vi "HOG Main.vi"() -> ()   [LabVIEW 2018]
doc: "This template is for the Queued Message Handler design pattern.\n\nThe Event Handling Loop generates messages based on user interface actions.\n\nThe Message Handling Loop processes messages generated by the Event Handling Loop, or by other messages. The messages are string values, so new messages can be added easily to the Message Cases case structure in the Message Handling Loop. Each message cluster can also provide an optional value for Message Data, which is a variant that can be converted to whatever message-specific data is required."
uses:
  controls/HOG UI Data.ctl
  <vilib>/GPower/Logger - Text/Library/Text Logger Class/Text Logger.lvclass
  C:/Program Files (x86)/National Instruments/LabVIEW 2018/vi.lib/GPower/Logger/Library/Logger Class/Logger.lvclass
  <vilib>/GPower/Dictionary/Library/Dictionary Class/Dictionary.lvclass
  support/Diploma Info.ctl
  <vilib>/Utility/sysdir.llb/System Directory Type.ctl
  <vilib>/GPower/Logger/Library/Logger Class/Logger.lvclass/Logger.ctl
  <vilib>/GPower/Array/Library/SearchMult/SearchMult1.vi
  8841ee87-444d-4723-9e2d-6f9928da492d.vi
  <vilib>/GPower/Logger/Library/Logger Class/Accessors/Get Enabled State.vi
  <vilib>/GPower/Logger/Library/Logger Class/Accessors/Get Severity Level Threshold.vi
  <vilib>/GPower/Logger/Library/Logger Class/Logger/Promote.vi
  <vilib>/GPower/Logger/Library/Logger Class/Accessors/Get Error And Warning Promotion.vi
  support/Message Queue/Enqueue Message (Single).vi
  <vilib>/GPower/Dictionary/Library/Dictionary Class/Get/Get Path.vi
  <vilib>/Utility/error.llb/Error Cluster From Error Code.vi
  <vilib>/GPower/UI/Library/Controls/Clear Control/Clear Listbox.vi
  <vilib>/GPower/UI/Library/Redraw/Defer Panel Updates (VI).vi
  <vilib>/GPower/UI/Library/Redraw/Undefer Panel Updates (VI).vi
  <vilib>/ErrorRing/Error Ring.xnode
  <vilib>/GPower/Logger/Library/Logger Class/Logger.lvclass
  support/Message Queue/HOG Message Queue.lvlib
  support/User Event - Stop/HOG User Event - Stop.lvlib
  <vilib>/GPower/UI/Library/GP UI.lvlib
  <vilib>/GPower/Array/GPArray.lvlib
  <vilib>/GPower/String/Library/GPString.lvlib
  <vilib>/Utility/NIReport.llb/NI_ReportGenerationCore.lvlib
  <vilib>/GPower/Files & Folders/Library/GPFilesFolders.lvlib
panel:
  in  "Tab Control":enum32{"Page 1", "Page 2", "Page 3"}(tab)
  in  "Load Event":bool
  in  "Event Folder Path":path
  in  "Manual":bool
  in  "MemberList":i32[](listbox)
  in  "Search":string
  out "Status":string
  in  "Cancel Print":bool
  in  "Print Button":bool
  in  "Help Radio Buttons":enum32{"Help", "No Help"}(radio) caption="Hjælpemiddel?"
  out "Diplom Navn":string
  out "Længde":string
  out "Diplom Pitcture":u16(ring)
  in  "Length Radio Buttons":enum32{"Baner", "Længde"}(radio)
  in  "Baner":u16
  in  "Navn":string
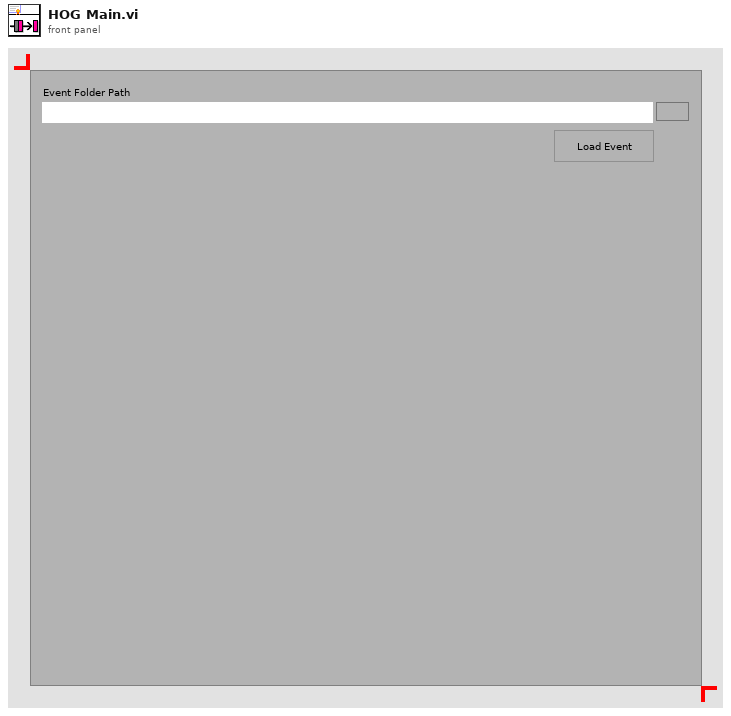
[diagram p1: front panel]
types:
  T1 = typedef "HOG UI Data.ctl" = cluster{"Status Ref":refnum<vi>, "Exit Button Ref":refnum<vi>, "Search Ref":refnum<vi>, "MemberList Ref":refnum<vi>, "This VI Ref":refnum<vi>, "Event Folder Path":path, "Load Event Ref":refnum<vi>, "Tab Control Ref":refnum<vi>, "Baner Ref":refnum<vi>, "Printer Name":string, "Diploma Template Path":path, "Text Logger":refnum<class "Text Logger.lvclass">}
  T2 = typedef "HOG Message Queue.lvlib/All Message Queues.ctl" = cluster{"UI":refnum<queue>, "Member":refnum<queue>}
  T3 = typedef "Diploma Info.ctl" = cluster{"Name":string, "Length Diploma":string, "Length":u16, "Help?":bool}
  T4 = typedef "System Directory Type.ctl" = i32
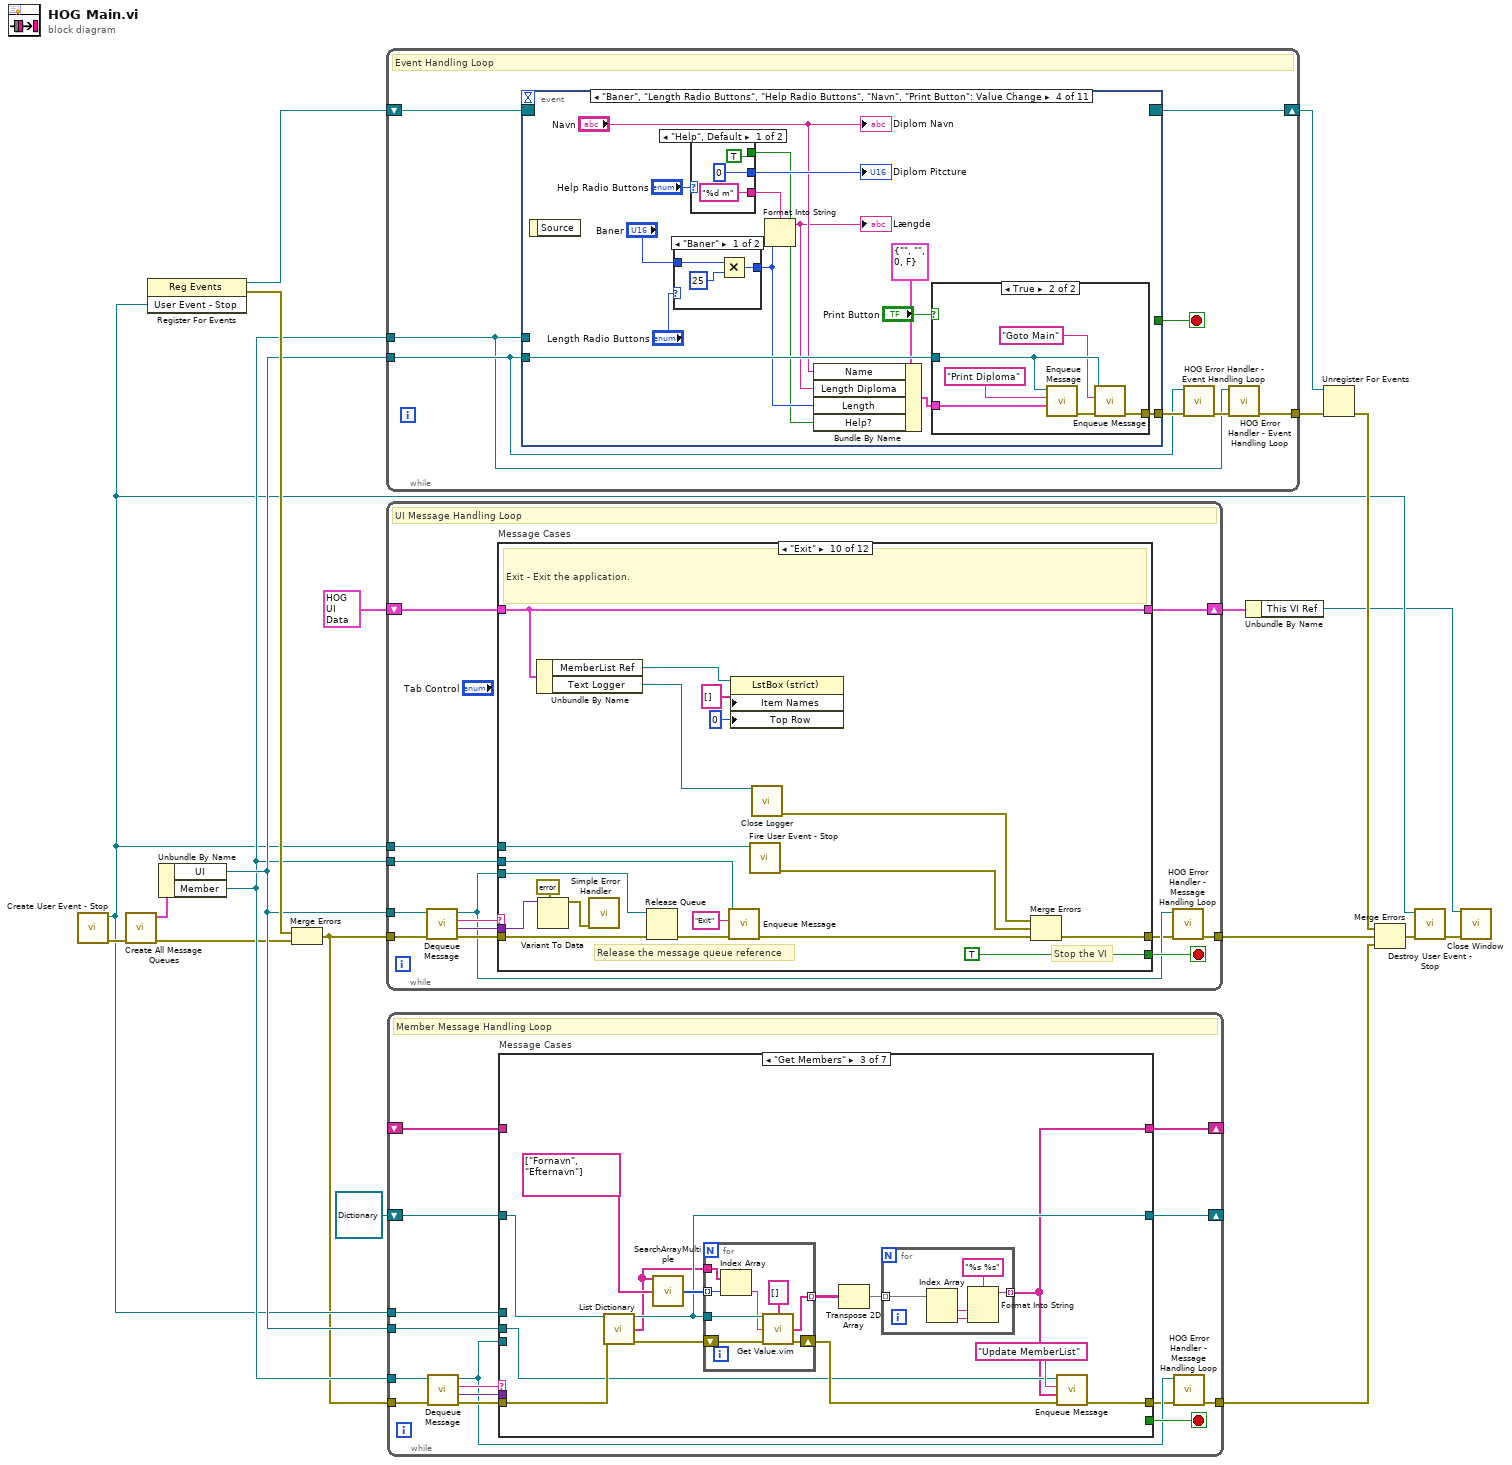
[diagram p0: block diagram]
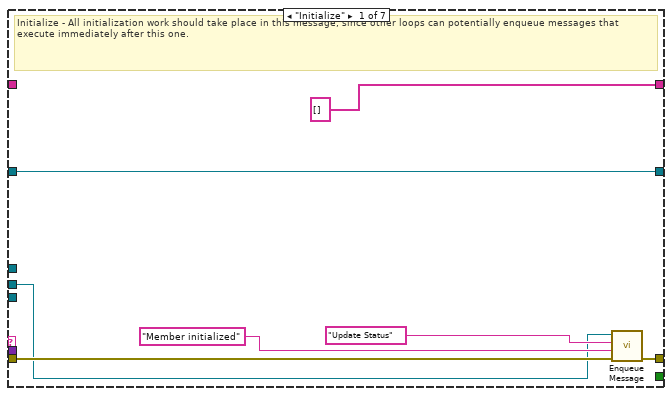
[diagram p2: hidden frame]
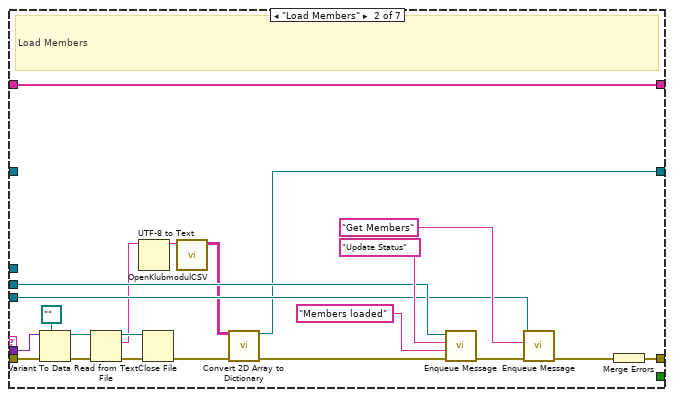
[diagram p3: hidden frame]
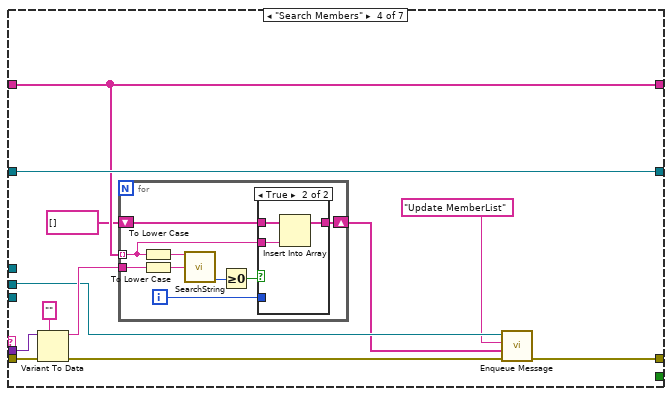
[diagram p4: hidden frame]
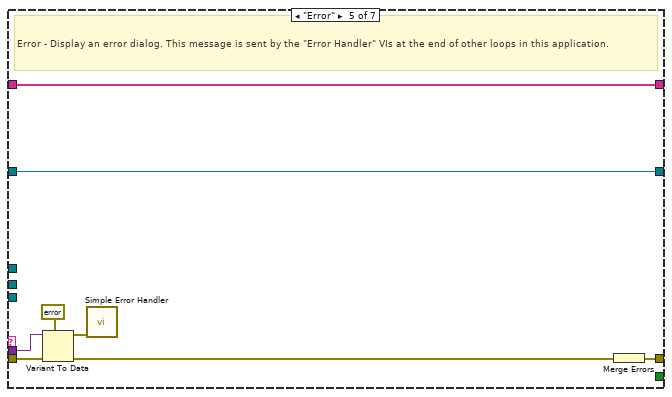
[diagram p6: hidden frame]
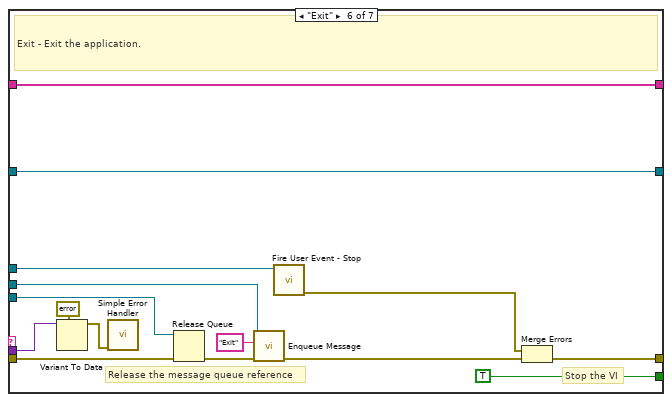
[diagram p7: hidden frame]
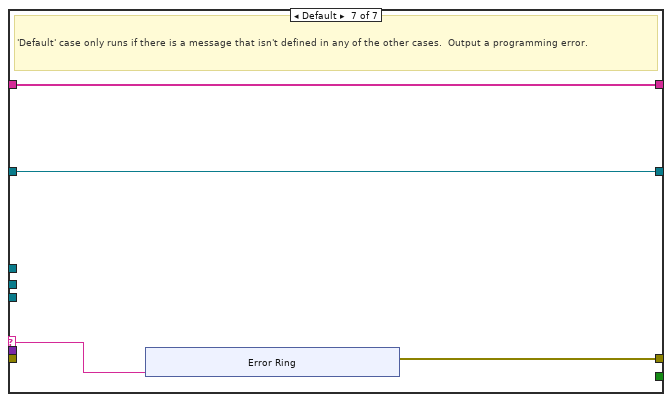
[diagram p8: hidden frame]
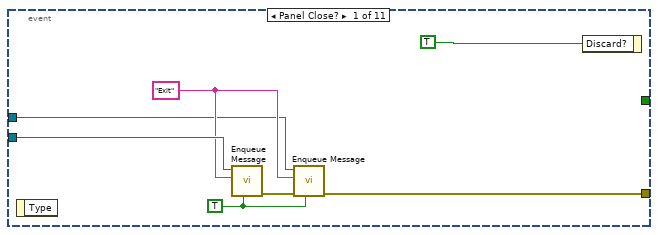
[diagram p9: hidden frame]
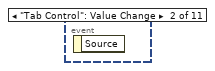
[diagram p10: hidden frame]
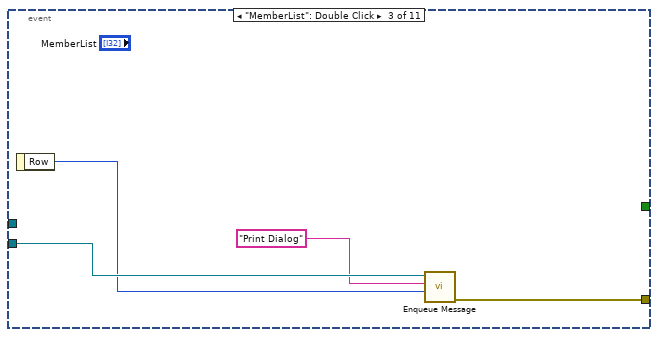
[diagram p11: hidden frame]
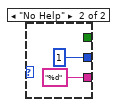
[diagram p14: hidden frame]
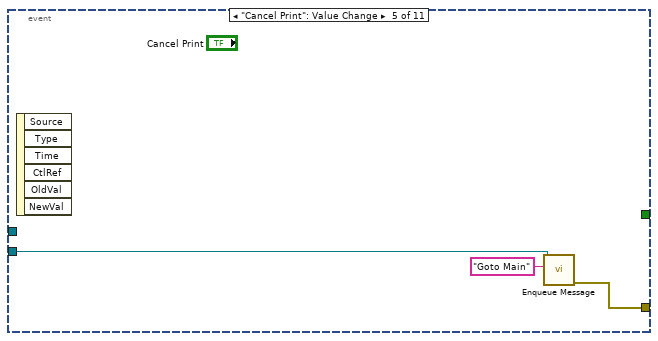
[diagram p15: hidden frame]
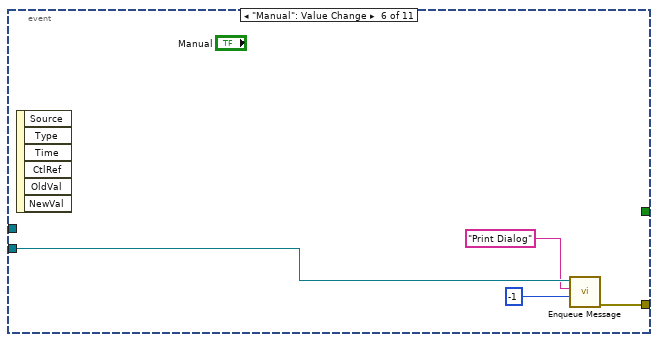
[diagram p16: hidden frame]
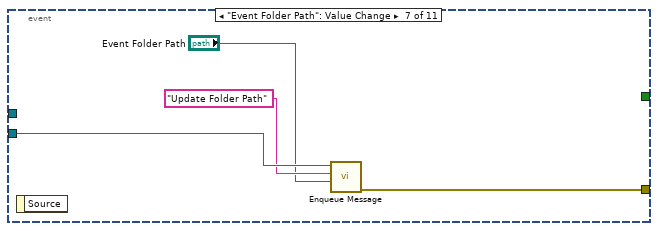
[diagram p17: hidden frame]
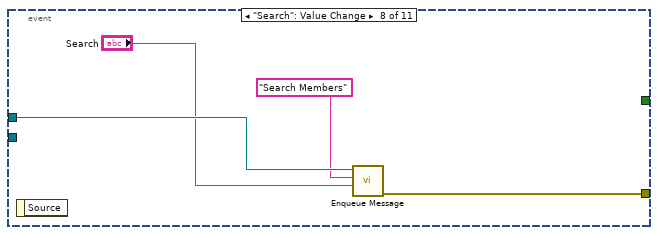
[diagram p18: hidden frame]
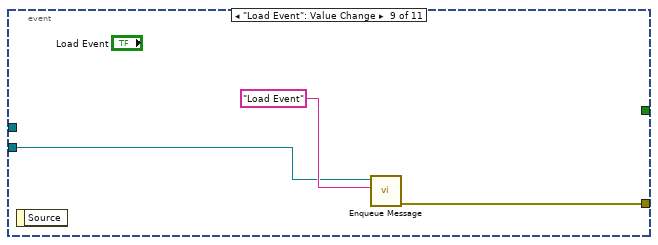
[diagram p19: hidden frame]
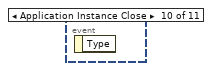
[diagram p20: hidden frame]
diagram:
  n1 = call "Create User Event - Stop.vi"() -> ("error out"=w18:errorcluster, "User Event - Stop"=w6:refnum<user-event>)  [unwired: 10 in]
  n2 = call "Create All Message Queues.vi"("error in (no error)"=w18) -> ("error out"=w5:errorcluster, "Message Queues out"=w20:T2)  [unwired: 9 in]
  n3 = register-events(w6) -> (reference out=w12:refnum<event-registration>, error out=w11:errorcluster)  [unwired: 2 in]
  n4 = Unbundle By Name(w20) -> ("UI"=w9:refnum<queue>, "Member"=w7:refnum<queue>)
  n5 = Merge Errors(w11, w5) -> (w4:errorcluster)
  n6 = while {
    tunnel: w9 -> [w22]
    shift-right: [w27] -> w15
    shift-left: w12 -> [w28]
    tunnel: [w23] -> w13
    tunnel: w7 -> [w21]
    stop <- w25 stop-if-true
    # "Event Handling Loop"
    n7 = event shown="[3] \"Baner\", \"Length Radio Buttons\", \"Help Radio Buttons\", \"Navn\", \"Print Button\": Value Change" {
      selector: w28 -> [_ _ _ _ _ _ _ _ _ _ _]
      dyn-events: [_ _ _ _ _ _ _ _ _ _ _] -> w27
      timeout: _ -> [_ _ _ _ _ _ _ _ _ _ _]
      tunnel: [_ _ _ _ _ _ _ _ _ _ TRUE ("Discard?")] -> w25
      tunnel: w22 -> [w34 _ w38 w50 w70 w74 w78 _ w84 _ _]
      tunnel: [w32 _ w39 w49 w71 w75 w79 w83 w86 _ _] -> w26
      tunnel: w21 -> [w30 _ _ _ _ _ _ w82 _ _ _]
      event Panel Close? {
        w29 = TRUE ("Priority Message? (F)")
        w31 = "Exit" ("Message")
        n8 = event-data() -> ()  [unwired: 1 in, 1 out]
        n9 = call-poly "Enqueue Message.vi"("Priority Message? (F)"=w29, "Message"=w31, "Message Queue"=w34) -> ("error out"=w33:errorcluster)  [unwired: 7 in, 1 out]
        n10 = call-poly "Enqueue Message.vi"("Priority Message? (F)"=w29, "error in (no error)"=w33, "Message"=w31, "Message Queue"=w30) -> ("error out"=w32:errorcluster)  [unwired: 6 in, 1 out]
        n11 = event-data("Discard?"=TRUE) -> ()  [unwired: 1 in, 1 out]
      }
      event "Tab Control": Value Change {
        n12 = event-data() -> ()  [unwired: 1 in, 1 out]
      }
      event "MemberList": Double Click {
        n13 = event-data() -> ("Row"=w36:i32)  [unwired: 1 in]
        n14 = call-poly "Enqueue Message.vi"("Message Data"=w36, "Message"="Print Dialog", "Message Queue"=w38) -> ("error out"=w39:errorcluster)  [unwired: 7 in, 1 out]
      }
      event "Baner", "Length Radio Buttons", "Help Radio Buttons", "Navn", "Print Button": Value Change {
        n15 = event-data() -> ()  [unwired: 1 in, 1 out]
        n16 = case shown="\"Baner\"" "Length Radio Buttons" {
          tunnel: "Baner" -> [w62 w63]
          tunnel: [w60 w63] -> w43
          frame "Baner" {
            n17 = Multiply(x=w62, y=u16 25) -> (x*y=w60:u16)
          }
          frame "Længde" {
          }
        }
        n18 = case shown="\"Help\", Default" "Help Radio Buttons" {
          tunnel: ["%d m" ("format string") "%d" ("format string")] -> w53
          tunnel: [u16 0 ("Diplom Pitcture") u16 1 ("Diplom Pitcture")] -> w52
          tunnel: [TRUE _] -> w41
          frame "Help", Default {
          }
          frame "No Help" {
          }
        }
        "Diplom Pitcture" <- w52
        n19 = Format Into String(format string=w53, w43) -> (resulting string=w44:string)  [unwired: 2 in, 1 out]
        "Længde" <- w44
        n20 = Bundle By Name(cluster=T3 {"Name"="", "Length Diploma"="", "Length"=0, "Help?"=FALSE}, "Name"="Navn", "Length Diploma"=w44, "Length"=w43, "Help?"=w41) -> (w42:T3)
        n21 = case shown="True" "Print Button" {
          tunnel: w50 -> [_ w55]
          tunnel: [_ w56] -> w49
          tunnel: w42 -> [_ w58]
          frame False {
          }
          frame True {
            n22 = call-poly "Enqueue Message.vi"("Message Data"=w58, "Message"="Print Diploma", "Message Queue"=w55) -> ("error out"=w57:errorcluster)  [unwired: 7 in, 1 out]
            n23 = call-poly "Enqueue Message.vi"("error in (no error)"=w57, "Message"="Goto Main", "Message Queue"=w55) -> ("error out"=w56:errorcluster)  [unwired: 7 in, 1 out]
          }
        }
        "Diplom Navn" <- "Navn"
      }
      event "Cancel Print": Value Change {
        n24 = event-data() -> ()  [unwired: 1 in, 6 out]
        n25 = call-poly "Enqueue Message.vi"("Message"="Goto Main", "Message Queue"=w70) -> ("error out"=w71:errorcluster)  [unwired: 8 in, 1 out]
      }
      event "Manual": Value Change {
        n26 = event-data() -> ()  [unwired: 1 in, 6 out]
        n27 = call-poly "Enqueue Message.vi"("Message Data"=-1, "Message"="Print Dialog", "Message Queue"=w74) -> ("error out"=w75:errorcluster)  [unwired: 7 in, 1 out]
      }
      event "Event Folder Path": Value Change {
        n28 = event-data() -> ()  [unwired: 1 in, 1 out]
        n29 = call-poly "Enqueue Message.vi"("Message Data"="Event Folder Path", "Message"="Update Folder Path", "Message Queue"=w78) -> ("error out"=w79:errorcluster)  [unwired: 7 in, 1 out]
      }
      event "Search": Value Change {
        n30 = event-data() -> ()  [unwired: 1 in, 1 out]
        n31 = call-poly "Enqueue Message.vi"("Message Data"="Search", "Message"="Search Members", "Message Queue"=w82) -> ("error out"=w83:errorcluster)  [unwired: 7 in, 1 out]
      }
      event "Load Event": Value Change {
        n32 = event-data() -> ()  [unwired: 1 in, 1 out]
        n33 = call-poly "Enqueue Message.vi"("Message"="Load Event", "Message Queue"=w84) -> ("error out"=w86:errorcluster)  [unwired: 8 in, 1 out]
      }
      event Application Instance Close {
        n34 = event-data() -> ()  [unwired: 1 in, 1 out]
      }
      event User Event {
        # "The Message Handling Loop processed an \"Exit\" message, which fired this event to stop the Event Handling Loop."
        n35 = event-data() -> ()  [unwired: 1 in, 1 out]
      }
    }
    n36 = call "HOG Error Handler - Event Handling Loop.vi"("error in (no error)"=w26, "Message Queue"=w22) -> ("dup error in"=w24:errorcluster)  [unwired: 8 in, 1 out]
    n37 = call "HOG Error Handler - Event Handling Loop.vi"("error in (no error)"=w24, "Message Queue"=w21) -> ("dup error in"=w23:errorcluster)  [unwired: 8 in, 1 out]
  }
  n38 = while {
    tunnel: w9 -> [w92]
    shift-right: [w99] -> w2
    shift-left: T1 {"Status Ref"=refnum, "Exit Button Ref"=refnum, "Search Ref"=refnum, "MemberList Ref"=refnum, "This VI Ref"=refnum, "Event Folder Path"=path "", "Load Event Ref"=refnum, "Tab Control Ref"=refnum, "Baner Ref"=refnum, "Printer Name"="", "Diploma Template Path"=path "", "Text Logger"=refnum} ("Data Cluster") -> [w100]
    tunnel: w6 -> [w97]
    tunnel: w4 -> [w96]
    tunnel: [w90] -> w19
    tunnel: w7 -> [w88]
    stop <- w98 stop-if-true
    # "UI Message Handling Loop"
    n39 = call "Dequeue Message.vi"("error in (no error)"=w96, "Message Queue"=w92) -> ("error out"=w95:errorcluster, "Message Data"=w93:variant, "Message"=w94:string, "dup Message Queue"=w91:refnum<queue>)  [unwired: 6 in]
    n40 = case "Message Cases" shown="\"Exit\"" w94 {
      selector: w94 -> [_ _ _ _ _ w173 _ _ _ _ w257 _]
      tunnel: w91 -> [w120 _ _ _ _ w168 _ w196 _ w256 _ _]
      tunnel: w95 -> [w105 w130 w136 w150 w157 w184 w195 w197 w237 w251 _ w269]
      tunnel: [w124 w131 w137 w149 w158 w169 w195 w211 w231 w254 w258 w270] -> w89
      tunnel: w100 -> [w106 w126 w138 w148 w161 w187 w194 w207 w236 w243 w259 w273]
      tunnel: [w123 w127 w138 w148 w161 w187 w194 w208 w236 w243 w259 w273] -> w99
      tunnel: [_ _ _ _ _ _ _ _ _ TRUE _ _] -> w98
      tunnel: w93 -> [_ w129 w135 w143 w156 w183 _ _ w235 w248 _ w271]
      tunnel: w97 -> [_ _ _ _ _ _ _ _ _ w253 _ _]
      tunnel: w88 -> [_ _ _ _ _ _ _ w210 _ w244 _ _]
      frame "Initialize" {
        w112 = T4 0 items=["User Home"=0, "User Desktop"=1, "User Documents"=2, "User Application Data"=3, "User Preferences"=4, "User Temporary"=5, "Public Documents"=6, "Public Application Data"=7, "Public Preferences"=8, "Public Cache"=13, "System Core Libraries"=9, "System Installed Libraries"=10, "Application Files"=11, "Boot Volume Root"=12] ("system directory type")
        # "Initialize - All initialization work should take place in this message, since other loops can potentially enqueue messages that execute immediately after this one."
        n41 = control-ref of="Tab Control"() -> (w108:refnum<vi>)
        n42 = control-ref of="Load Event"() -> (w113:refnum<vi>)
        n43 = control-ref of="MemberList"() -> (w101:refnum<vi>)
        n44 = control-ref of="This VI"() -> (w102:refnum<vi>)
        n45 = control-ref of="Baner"() -> (w109:refnum<vi>)
        n46 = control-ref of="Search"() -> (w118:refnum<vi>)
        n47 = control-ref of="Status"() -> (w122:refnum<vi>)
        n48 = control-ref of="Event Folder Path"() -> (w111:refnum<vi>)
        n49 = call <vilib>:"Get System Directory.vi"("system directory type"=w112) -> ("system directory"=w110:path)  [unwired: 10 in]
        n50 = call-poly <vilib>:"Clear Control.vi"("Listbox"=w101, "Error in"=w105) -> ("Error out"=w117:errorcluster)  [unwired: 13 in]
        n51 = call <vilib>:"Fit Front Panel By Markers.vi"("VI Refnum"=w102, "Error in"=w117) -> ("Error out"=w116:errorcluster)  [unwired: 13 in]
        n52 = call <vilib>:"Set Standard Window.vi"("VI Refnum"=w102, "Error in"=w116) -> ("Error out"=w104:errorcluster)  [unwired: 13 in]
        n53 = call <vilib>:"Center On Monitor.vi"("VI Refnum"=w102, "Error in"=w104) -> ("Error out"=w103:errorcluster)  [unwired: 13 in]
        n54 = property class="VI"(reference=w102, error in=w103, "Front Panel.Title"="HOG Diplom" ("VI Name")) -> (error out=w114:errorcluster)  [unwired: 1 out]
        n55 = Bundle By Name(cluster=w106, "Search Ref"=w118, "MemberList Ref"=w101, "Status Ref"=w122, "This VI Ref"=w102, "Load Event Ref"=w113, "Tab Control Ref"=w108, "Baner Ref"=w109, "Event Folder Path"=w110) -> (w123:T1)
        n56 = property class="TabCtl (strict)"(reference=w108, "Value"=enum32{"Page 1", "Page 2", "Page 3"}."Page 1") -> ()  [unwired: 1 in, 2 out]
        n57 = property class="Path"(reference=w111, "Value"=w110) -> ()  [unwired: 1 in, 2 out]
        n58 = call-poly "Enqueue Message.vi"("error in (no error)"=w114, "Message Data"="UI Initialized" ("Initial Message"), "Message"="Update Status", "Message Queue"=w120) -> ("error out"=w124:errorcluster)  [unwired: 6 in, 1 out]
      }
      frame "Update Folder Path" {
        n59 = Variant To Data(error in=w130, type=path "", Variant=w129) -> (data=w125:path, error out=w131:errorcluster)
        n60 = Bundle By Name(cluster=w126, "Event Folder Path"=w125) -> (w127:T1)
      }
      frame "Update Status" {
        # "Update Display - Convert the message data to a string to display in the Data Display indicator."
        n61 = Variant To Data(error in=w136, type="", Variant=w135) -> (data=→"Status":string, error out=w133:errorcluster)
        n62 = Merge Errors(w133) -> (w137:errorcluster)
      }
      frame "Update MemberList" {
        n63 = Unbundle By Name(w148) -> ("MemberList Ref"=w146:refnum<vi>, "This VI Ref"=w147:refnum<vi>)
        n64 = call-poly <vilib>:"Defer Panel Updates.vi"("VI Refnum"=w147, "Error in"=w150) -> ("Error out"=w145:errorcluster)  [unwired: 13 in]
        n65 = Variant To Data(error in=w145, type=string[] [] ("Item Names"), Variant=w143) -> (data=w140:string[], error out=w142:errorcluster)
        n66 = property class="LstBox (strict)"(reference=w146, error in=w142, "Item Names"=w140, "Top Row"=0 ("Focus Row")) -> (error out=w141:errorcluster)  [unwired: 1 out]
        n67 = call-poly <vilib>:"Undefer Panel Updates.vi"("VI Refnum"=w147, "Error in"=w141) -> ("Error out"=w149:errorcluster)  [unwired: 13 in]
      }
      frame "Print Dialog" {
        n68 = Unbundle By Name(w161) -> ("Tab Control Ref"=w160:refnum<vi>, "MemberList Ref"=w154:refnum<vi>)
        n69 = Variant To Data(error in=w157, type=0, Variant=w156) -> (data=w152:i32, error out=w158:errorcluster)
        n70 = Greater Or Equal To 0?(x=w152) -> (x >= 0?=w151:bool)
        n71 = case "Valid Index?" shown="True" w151 {
          tunnel: w154 -> [_ w165]
          tunnel: w152 -> [_ w163]
          tunnel: [_ w162] -> w153
          frame False {
          }
          frame True {
            n72 = property class="LstBox (strict)"(reference=w165) -> ("Item Names"=w164:string[])  [unwired: 1 in, 2 out]
            n73 = Index Array(array=w164, index=w163) -> (element=w162:string)
          }
        }
        n74 = property class="TabCtl (strict)"(reference=w160, "Value"=enum32{"Page 1", "Page 2", "Page 3"}."Page 3") -> ()  [unwired: 1 in, 2 out]
        n75 = property on="Navn" class="Str"("Val(Sgnl)"=w153) -> ()  [unwired: 2 in, 2 out]
      }
      frame "Print Diploma" {
        n76 = Unbundle By Name(w187) -> ("Printer Name"=w186:string, "Diploma Template Path"=w185:path, "Text Logger"=w180:refnum<class "Text Logger.lvclass">)
        n77 = Variant To Data(error in=w184, type=T3 {"Name"="", "Length Diploma"="", "Length"=0, "Help?"=FALSE}, Variant=w183) -> (data=w178:T3, error out=w182:errorcluster)
        n78 = Unbundle By Name(w178) -> ("Name"=w177:string, "Length Diploma"=w176:string, "Length"=w175:u16, "Help?"=w172:bool)
        n79 = call <vilib>:"BoolToTrueFalse.vi"("Boolean"=w172) -> ("String"=w171:string)
        n80 = Format Into String(format string="%s - %d - Help:%s", w177, w175, w171) -> (resulting string=w166:string)  [unwired: 2 in, 1 out]
        n81 = call <vilib>:"Log.vi"("Logger in"=w180, "Source"=w173, "Message"=w166, "Error in"=w182) -> ("Error out"=w181:errorcluster)  [unwired: 10 in, 1 out]
        n82 = call "Print Diploma.vi"("Length Diploma"=w176, "error in (no error)"=w181, "Name"=w177, "Printer Name"=w186, "Diploma Template Path"=w185) -> ("error out"=w170:errorcluster)  [unwired: 6 in]
        n83 = call-poly "Enqueue Message.vi"("error in (no error)"=w170, "Message Data"=w166, "Message"="Update Status", "Message Queue"=w168) -> ("error out"=w169:errorcluster)  [unwired: 6 in, 1 out]
      }
      frame "Goto Main" {
        n84 = Unbundle By Name(w194) -> ("Tab Control Ref"=w193:refnum<vi>, "Search Ref"=w191:refnum<vi>, "MemberList Ref"=w189:refnum<vi>)
        n85 = property class="TabCtl (strict)"(reference=w193, "Value"=enum32{"Page 1", "Page 2", "Page 3"}."Page 2") -> ()  [unwired: 1 in, 2 out]
        n86 = property class="LstBox (strict)"(reference=w189, "Top Row"=0) -> ()  [unwired: 1 in, 2 out]
        n87 = property class="Str"(reference=w191, "Value"="") -> ()  [unwired: 1 in, 2 out]
      }
      frame "Load Event" {
        n88 = Unbundle By Name(w207) -> ("Event Folder Path"=w204:path)
        n89 = Build Path(base path=w204, name or relative path="Diplom.dotx") -> (appended path=w202:path)
        n90 = Build Path(base path=w204, name or relative path="Members.csv") -> (appended path=w203:path)
        n91 = Build Path(base path=w204, name or relative path="Log.txt") -> (appended path=w198:path)
        n92 = call <vilib>:"Is Existing File.vi"("File Path"=w202) -> ("Existing File?"=w200:bool)  [unwired: 4 in]
        n93 = call <vilib>:"Is Existing File.vi"("File Path"=w203) -> ("Existing File?"=w201:bool)  [unwired: 4 in]
        n94 = And(x=w201, y=w200) -> (x .and. y?=w199:bool)
        n95 = case "File found?" shown="True" w199 {
          tunnel: [w212 w217] -> w211
          tunnel: w210 -> [_ w230]
          tunnel: [w214 w228] -> w208
          tunnel: w207 -> [w214 w227]
          tunnel: w203 -> [_ w226]
          tunnel: w202 -> [_ w225]
          tunnel: w198 -> [_ w222]
          tunnel: w197 -> [w212 w221]
          tunnel: w196 -> [_ w215]
          frame False {
            n96 = One Button Dialog(message="Vælg event folder") -> ()  [unwired: 1 in, 1 out]
          }
          frame True {
            n97 = call <vilib>:"New Text Logger.vi"("Log File Path"=w222, "Error in"=w221) -> ("Text Logger"=w220:refnum<class "Text Logger.lvclass">, "Error out"=w219:errorcluster)  [unwired: 12 in]
            n98 = call <vilib>:"Query Available Printers.vi"("error in (no error)"=w219) -> ("error out"=w224:errorcluster, "default printer"=w223:string)  [unwired: 8 in, 1 out]
            n99 = Bundle By Name(cluster=w227, "Printer Name"=w223, "Diploma Template Path"=w225, "Text Logger"=w220) -> (w228:T1)
            n100 = call-poly "Enqueue Message.vi"("error in (no error)"=w224, "Message Data"=w226, "Message"="Load Members", "Message Queue"=w230) -> ("error out"=w218:errorcluster)  [unwired: 6 in, 1 out]
            n101 = call-poly "Enqueue Message.vi"("error in (no error)"=w218, "Message"="Goto Main", "Message Queue"=w215) -> ("error out"=w217:errorcluster)  [unwired: 7 in, 1 out]
          }
        }
      }
      frame "Error" {
        # "Error - Display an error dialog. This message is sent by the \"Error Handler\" VIs at the end of other loops in this application."
        n102 = Variant To Data(error in=w237, type=errorcluster {"status"=FALSE, "code"=0, "source"=""} ("error constant"), Variant=w235) -> (data=w233:errorcluster, error out=w232:errorcluster)
        n103 = call <vilib>:"Simple Error Handler.vi"("error in (no error)"=w233) -> ()  [unwired: 4 in, 5 out]
        n104 = Merge Errors(w232) -> (w231:errorcluster)
      }
      frame "Exit" {
        # "Stop the VI"
        # "Release the message queue reference"
        # "Exit - Exit the application."
        n105 = Unbundle By Name(w243) -> ("MemberList Ref"=w240:refnum<vi>, "Text Logger"=w242:refnum<class "Text Logger.lvclass">)
        n106 = Variant To Data(type=errorcluster {"status"=FALSE, "code"=0, "source"=""} ("error constant"), Variant=w248) -> (data=w249:errorcluster)  [unwired: 1 in, 1 out]
        n107 = call <vilib>:"Simple Error Handler.vi"("error in (no error)"=w249) -> ()  [unwired: 4 in, 5 out]
        n108 = Release Queue(queue=w256, error in (no error)=w251) -> (error out=w246:errorcluster)  [unwired: 1 in, 2 out]
        n109 = call-poly "Enqueue Message.vi"("error in (no error)"=w246, "Message"="Exit", "Message Queue"=w244) -> ("error out"=w245:errorcluster)  [unwired: 7 in, 1 out]
        n110 = property class="LstBox (strict)"(reference=w240, "Item Names"=string[] [], "Top Row"=0) -> ()  [unwired: 1 in, 2 out]
        n111 = call "Fire User Event - Stop.vi"("User Event - Stop"=w253) -> ("error out"=w252:errorcluster)  [unwired: 10 in]
        n112 = call-dynamic "Close Logger.vi"("Logger"=w242) -> ("Error out"=w241:errorcluster)  [unwired: 14 in]
        n113 = Merge Errors(w241, w252, w245) -> (w254:errorcluster)
      }
      frame Default {
        # "'Default' case only runs if there is a message that isn't defined in any of the other cases.  Output a programming error."
        n114 = xnode "Error Ring"("parameter 0"=w257) -> ("error out"=w258:errorcluster)
      }
      frame "Set Caption" {
        n115 = Unbundle By Name(w273) -> ("Baner Ref"=w272:refnum<vi>)
        n116 = Variant To Data(error in=w269, type="", Variant=w271) -> (data=w267:string, error out=w270:errorcluster)
        n117 = property class="DigNum (strict)"(reference=w272, "Caption.Text"=w267) -> ()  [unwired: 1 in, 2 out]
      }
    }
    n118 = call "HOG Error Handler - Message Handling Loop.vi"("error in (no error)"=w89, "Message Queue"=w91) -> ("dup error in"=w90:errorcluster)  [unwired: 8 in, 1 out]
  }
  n119 = while {
    tunnel: w7 -> [w280]
    shift-right: [w287] -> _
    shift-left: refnum<class "Dictionary.lvclass"> refnum ("New Dictionary") -> [w288]
    tunnel: w6 -> [w285]
    tunnel: w4 -> [w284]
    tunnel: [w278] -> w10
    tunnel: w9 -> [w276]
    shift-right: [w275] -> _
    shift-left: _ -> [w274]
    stop <- w286 stop-if-true
    # "Member Message Handling Loop"
    n120 = call "Dequeue Message.vi"("error in (no error)"=w284, "Message Queue"=w280) -> ("error out"=w283:errorcluster, "Message Data"=w281:variant, "Message"=w282:string, "dup Message Queue"=w279:refnum<queue>)  [unwired: 6 in]
    n121 = case "Message Cases" shown="\"Get Members\"" w282 {
      selector: w282 -> [_ _ _ _ _ _ w394]
      tunnel: w279 -> [_ w303 _ _ _ w392 _]
      tunnel: w283 -> [w294 w315 w330 w353 w377 w389 _]
      tunnel: [w295 w317 w323 w349 w371 w383 w395] -> w277
      tunnel: w288 -> [w291 _ w331 w356 w376 w391 w396]
      tunnel: [w291 w299 w327 w356 w376 w391 w396] -> w287
      tunnel: [_ _ _ _ _ TRUE _] -> w286
      tunnel: w281 -> [_ w316 _ w354 w375 w386 _]
      tunnel: w285 -> [_ _ _ _ _ w385 _]
      tunnel: w276 -> [w290 w307 w321 w348 _ w380 _]
      tunnel: [string[] [] w296 w319 w355 w370 w378 w393] -> w275
      tunnel: w274 -> [_ w296 _ w355 w370 w378 w393]
      frame "Initialize" {
        # "Initialize - All initialization work should take place in this message, since other loops can potentially enqueue messages that execute immediately after this one."
        n122 = call-poly "Enqueue Message.vi"("error in (no error)"=w294, "Message Data"="Member initialized" ("Initial Message"), "Message"="Update Status", "Message Queue"=w290) -> ("error out"=w295:errorcluster)  [unwired: 6 in, 1 out]
      }
      frame "Load Members" {
        # "Load Members"
        n123 = Variant To Data(error in=w315, type=path "", Variant=w316) -> (data=w312:path, error out=w313:errorcluster)
        n124 = Read from Text File(file (use dialog)=w312, error in=w313) -> (refnum out=w310:refnum<file>, text=w302:string, error out=w311:errorcluster)  [unwired: 2 in, 1 out]
        n125 = UTF-8 to Text(11:w302) -> (3:w301:string)  [unwired: 2 in, 1 out]
        n126 = Close File(refnum=w310, error in=w311) -> (error out=w298:errorcluster)  [unwired: 1 out]
        n127 = call "OpenKlubmodulCSV.vi"("CSV String"=w301) -> ("CSV Data"=w300:string[][])  [unwired: 10 in]
        n128 = call "Convert 2D Array to Dictionary.vi"("CSV Data"=w300, "Error in"=w298) -> ("Dictionary out"=w299:refnum<class "Dictionary.lvclass">, "Error out"=w297:errorcluster)  [unwired: 11 in, 1 out]
        n129 = call-poly "Enqueue Message.vi"("error in (no error)"=w297, "Message Data"="Members loaded" ("Message"), "Message"="Update Status", "Message Queue"=w307) -> ("error out"=w306:errorcluster)  [unwired: 6 in, 1 out]
        n130 = call-poly "Enqueue Message.vi"("error in (no error)"=w306, "Message"="Get Members", "Message Queue"=w303) -> ("error out"=w305:errorcluster)  [unwired: 7 in, 1 out]
        n131 = Merge Errors(w305) -> (w317:errorcluster)
      }
      frame "Get Members" {
        n132 = call <vilib>:"List Dictionary.vi"("Dictionary in"=w331, "Error in"=w330) -> ("Dictionary out"=w327:refnum<class "Dictionary.lvclass">, "Keys"=w326:string[], "Error out"=w325:errorcluster)  [unwired: 11 in]
        n133 = call-poly <vilib>:"SearchArrayMultiple.vi"("Array"=w326, "Elements to search for"=string[] ["Fornavn", "Efternavn"]) -> ("Indices of elements"=w328:i32[])  [unwired: 12 in, 1 out]
        n134 = for {
          tunnel: w328 -> [w343] mode=indexing
          tunnel: w326 -> [w344]
          tunnel: w327 -> [w342]
          shift-right: [w339] -> w324
          shift-left: w325 -> [w340]
          tunnel: [w337] -> w320 mode=indexing
          n135 = Index Array(array=w344, index=w343) -> (element=w341:string)
          n136 = call "Get Value.vim"("Dictionary in"=w342, "Value Type"=string[] [], "Key Path"=w341, "Error in"=w340) -> ("Value"=w337:string[], "Error out"=w339:errorcluster)  [unwired: 9 in, 1 out]
        }
        n137 = Transpose 2D Array(2D array=w320) -> (transposed array=w318:string[][])
        n138 = for {
          tunnel: w318 -> [w336] mode=indexing
          tunnel: [w333] -> w319 mode=indexing
          n139 = Index Array(array=w336) -> (element #1=w335:string, element #2=w334:string)  [unwired: 2 in]
          n140 = Format Into String(format string="%s %s", w335, w334) -> (resulting string=w333:string)  [unwired: 2 in, 1 out]
        }
        n141 = call-poly "Enqueue Message.vi"("error in (no error)"=w324, "Message Data"=w319, "Message"="Update MemberList", "Message Queue"=w321) -> ("error out"=w323:errorcluster)  [unwired: 6 in, 1 out]
      }
      frame "Search Members" {
        n142 = Variant To Data(error in=w353, type="", Variant=w354) -> (data=w351:string, error out=w350:errorcluster)
        n143 = for {
          tunnel: w351 -> [w361]
          shift-right: [w362] -> w346
          shift-left: string[] [] -> [w363]
          tunnel: w355 -> [w357] mode=indexing
          i -> [w358]
          n144 = To Lower Case(string=w357) -> (all lower case string=w359:string)
          n145 = To Lower Case(string=w361) -> (all lower case string=w360:string)
          n146 = call <vilib>:"SearchString.vi"("String"=w359, "Search string"=w360) -> ("Offset past match"=w365:i32)  [unwired: 11 in, 2 out]
          n147 = Greater Or Equal To 0?(x=w365) -> (x >= 0?=w364:bool)
          n148 = case shown="True" w364 {
            tunnel: w363 -> [w366 w369]
            tunnel: [w366 w368] -> w362
            tunnel: w358 -> [_ _]
            tunnel: w357 -> [_ w367]
            frame False {
            }
            frame True {
              n149 = Insert Into Array(array=w369, new element=w367) -> (w368:string[])  [unwired: 1 in]
            }
          }
        }
        n150 = call-poly "Enqueue Message.vi"("error in (no error)"=w350, "Message Data"=w346, "Message"="Update MemberList", "Message Queue"=w348) -> ("error out"=w349:errorcluster)  [unwired: 6 in, 1 out]
      }
      frame "Error" {
        # "Error - Display an error dialog. This message is sent by the \"Error Handler\" VIs at the end of other loops in this application."
        n151 = Variant To Data(error in=w377, type=errorcluster {"status"=FALSE, "code"=0, "source"=""} ("error constant"), Variant=w375) -> (data=w373:errorcluster, error out=w372:errorcluster)
        n152 = call <vilib>:"Simple Error Handler.vi"("error in (no error)"=w373) -> ()  [unwired: 4 in, 5 out]
        n153 = Merge Errors(w372) -> (w371:errorcluster)
      }
      frame "Exit" {
        # "Stop the VI"
        # "Release the message queue reference"
        # "Exit - Exit the application."
        n154 = Variant To Data(type=errorcluster {"status"=FALSE, "code"=0, "source"=""} ("error constant"), Variant=w386) -> (data=w387:errorcluster)  [unwired: 1 in, 1 out]
        n155 = call <vilib>:"Simple Error Handler.vi"("error in (no error)"=w387) -> ()  [unwired: 4 in, 5 out]
        n156 = Release Queue(queue=w392, error in (no error)=w389) -> (error out=w382:errorcluster)  [unwired: 1 in, 2 out]
        n157 = call-poly "Enqueue Message.vi"("error in (no error)"=w382, "Message"="Exit", "Message Queue"=w380) -> ("error out"=w381:errorcluster)  [unwired: 7 in, 1 out]
        n158 = call "Fire User Event - Stop.vi"("User Event - Stop"=w385) -> ("error out"=w384:errorcluster)  [unwired: 10 in]
        n159 = Merge Errors(w384, w381) -> (w383:errorcluster)
      }
      frame Default {
        # "'Default' case only runs if there is a message that isn't defined in any of the other cases.  Output a programming error."
        n160 = xnode "Error Ring"("parameter 0"=w394) -> ("error out"=w395:errorcluster)
      }
    }
    n161 = call "HOG Error Handler - Message Handling Loop.vi"("error in (no error)"=w277, "Message Queue"=w279) -> ("dup error in"=w278:errorcluster)  [unwired: 8 in, 1 out]
  }
  n162 = Unbundle By Name(w2) -> ("This VI Ref"=w1:refnum<vi>)
  n163 = Unregister For Events(event registration refnum=w15, error in=w13) -> (error out=w16:errorcluster)
  n164 = Merge Errors(w16, w19, w10) -> (w17:errorcluster)
  n165 = call "Destroy User Event - Stop.vi"("error in (no error)"=w17, "User Event - Stop"=w6) -> ("error out"=w3:errorcluster)  [unwired: 9 in]
  n166 = call <vilib>:"Close Window.vi"("VI Refnum"=w1, "Error in"=w3) -> ()  [unwired: 13 in, 1 out]
